vi "Get Buttons Reference.vi"(8 "error in (no error)":errorcluster, 10 "VI reference (calling)":refnum<vi>, 11 "Dialog in":refnum<class "Dialog.lvclass">) -> (0 "error out":errorcluster, 2 "VI reference (dup)":refnum<vi>, 3 "Dialog out":refnum<class "Dialog.lvclass">)   [LabVIEW 2012, in "Dialog.lvlib" / "Dialog.lvclass"]
uses:
  Dialog.lvclass
  Dialog.lvclass/Dialog.ctl
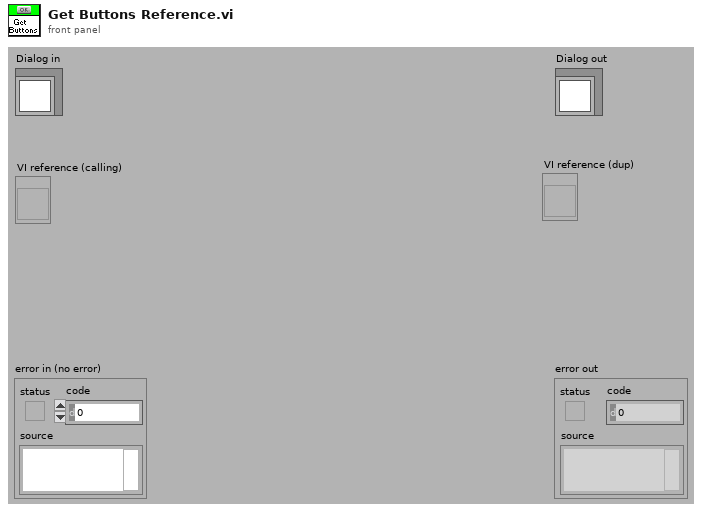
[diagram p1: front panel]
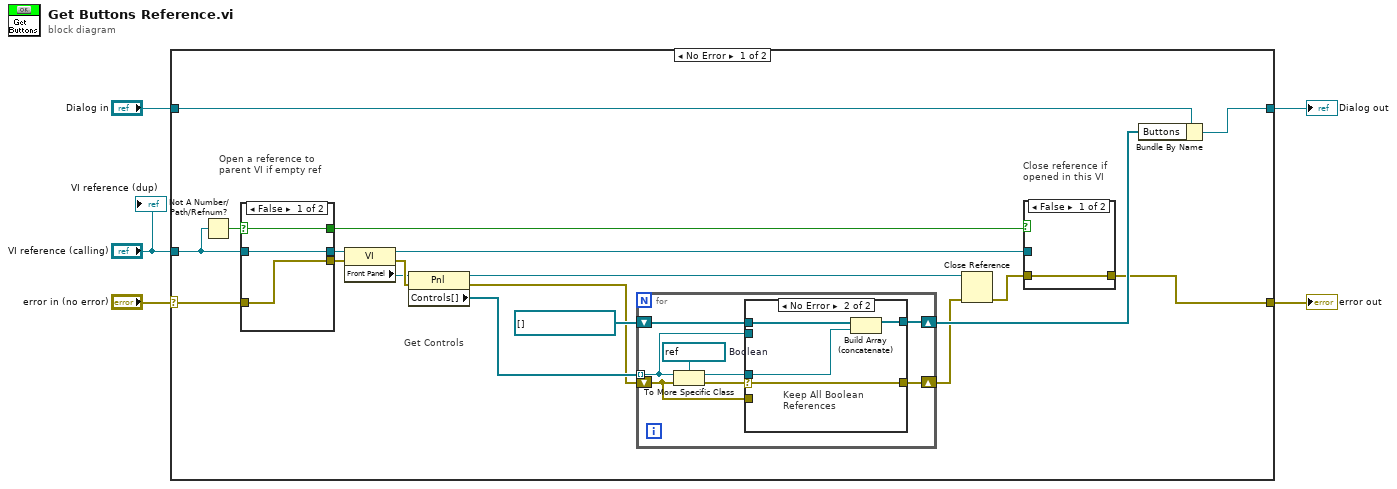
[diagram p0: block diagram]
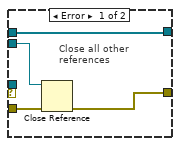
[diagram p2: hidden frame]
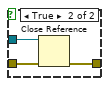
[diagram p3: hidden frame]
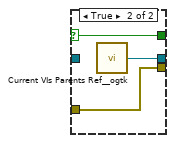
[diagram p4: hidden frame]
diagram:
  n1 = case shown="No Error" "error in (no error)" {
    selector: "error in (no error)" -> [w17 w52]
    tunnel: [w7 w52] -> w4
    tunnel: [w21 w51] -> w2
    tunnel: "Dialog in" -> [w22 w51]
    tunnel: "VI reference (calling)" -> [w18 _]
    frame No Error {
      # "Get Controls"
      # "Close reference if\nopened in this VI"
      # "Open a reference to\nparent VI if empty ref"
      n2 = Not A Number/Path/Refnum?(number/path/refnum=w18) -> (NaN/Path/Refnum?=w20:bool)
      n3 = case shown="False" w20 {
        selector: w20 -> [w46 w50]
        tunnel: [w46 w50] -> w15
        tunnel: [w47 w49] -> w19
        tunnel: w18 -> [w47 _]
        tunnel: w17 -> [w45 w48]
        tunnel: [w45 w48] -> w16
        frame False {
        }
        frame True {
          n4 = call <userlib>:"Current VIs Parents Ref__ogtk.vi"() -> ("Calling VI's Reference"=w49:refnum<vi>)  [unwired: 2 out]
        }
      }
      n5 = property on="Property Node" class="VI"(reference=w19, error in=w16) -> (reference out=w14:refnum<vi>, error out=w24:errorcluster, "Front Panel"=w23:refnum<vi>)
      n6 = property on="Property Node" class="Pnl"(reference=w23, error in=w24) -> (reference out=w13:refnum<vi>, error out=w6:errorcluster, "Controls[]"=w11:refnum<vi>[])
      n7 = for {
        tunnel: w11 -> [w25] mode=indexing
        shift-right: [w32] -> w10
        shift-left: refnum<vi>[] [] -> [w31]
        shift-right: [w30] -> w8
        shift-left: w6 -> [w26]
        w29 = refnum<vi> refnum  # Boolean
        n8 = To More Specific Class(target class=w29, reference=w25, error in=w26) -> (specific class reference=w27:refnum<vi>, error out=w28:errorcluster)
        n9 = case shown="No Error" w28 {
          selector: w28 -> [_ w37]
          tunnel: w27 -> [_ w38]
          tunnel: [w36 w39] -> w32
          tunnel: w31 -> [w36 w40]
          tunnel: [w34 w37] -> w30
          tunnel: w26 -> [w35 _]
          tunnel: w25 -> [w33 _]
          frame Error {
            # "Close all other\nreferences"
            n10 = Close Reference(reference=w33, error in (no error)=w35) -> (error out=w34:errorcluster)
          }
          frame No Error {
            # "Keep All Boolean\nReferences"
            n11 = Build Array (concatenate)(w40, w38) -> (w39:refnum<vi>[])
          }
        }
      }
      n12 = Close Reference(reference=w13, error in (no error)=w8) -> (error out=w12:errorcluster)
      n13 = case shown="False" w15 {
        tunnel: w14 -> [_ w44]
        tunnel: [w41 w43] -> w7
        tunnel: w12 -> [w41 w42]
        frame False {
        }
        frame True {
          n14 = Close Reference(reference=w44, error in (no error)=w42) -> (error out=w43:errorcluster)
        }
      }
      n15 = Bundle By Name(cluster=w22, "Buttons"=w10) -> (w21:refnum<class "Dialog.lvclass">)
    }
    frame Error {
    }
  }
  "error out" <- w4
  "Dialog out" <- w2
  "VI reference (dup)" <- "VI reference (calling)"
